vi "TimeForVIPCheck.vi"(8 "error in (no error)":errorcluster) -> (0 "error out":errorcluster, 3 "Check VIP?":bool)   [LabVIEW 2014, in "Raspberry Pi Compatible Compiler for LabVIEW.lvlib" / "GitHub API.lvlib"]
uses:
  GitHub API.lvlib
  RasPi Compiler/Compile and Download App/Custom Controls/Local Setup Parameters.ctl
  Raspberry Pi Compatible Compiler for LabVIEW.lvlib
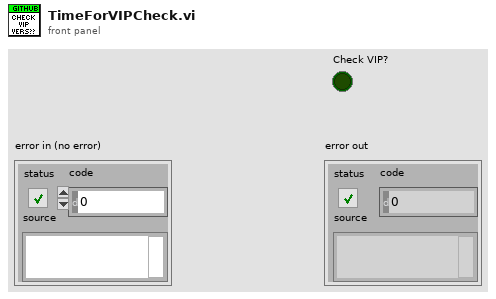
[diagram p1: front panel]
types:
  T1 = typedef "Raspberry Pi Compatible Compiler for LabVIEW.lvlib/Local Setup Parameters.ctl" = enum16{"Add Last VI", "Read Last VI", "Add Board IP", "Remove Board IP", "Read All Board IP", "Add Runtime Version", "Read Runtime Version", "Add Package Version", "Read Package Version", "Add VIPCheck Time", "Read VIPCheck Time"}
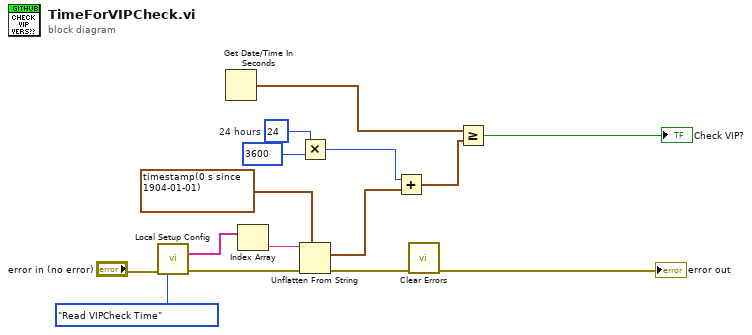
[diagram p0: block diagram]
diagram:
  w1 = 24  # 24 hours
  n1 = call "Local Setup Config.vi"("Local Setup Param"=Local_Setup_Parameters."Read VIPCheck Time", "error in"="error in (no error)") -> ("KeyValues"=w13:string[], "error out"=w12:errorcluster)  [unwired: 10 in, 2 out]
  n2 = Get Date/Time In Seconds() -> (seconds since 1Jan1904=w5:timestamp)
  n3 = Index Array(array=w13) -> (element=w11:string)  [unwired: 1 in]
  n4 = Multiply(x=w1, y=3600) -> (x*y=w2:i32)
  n5 = Unflatten From String(type=timestamp(0 s since 1904-01-01) ("Time Stamp"), binary string=w11, error in (no error)=w12) -> (value=w7:timestamp, error out=w9:errorcluster)  [unwired: 2 in, 1 out]
  n6 = Add(x=w2, y=w7) -> (x+y=w4:timestamp)
  n7 = call <vilib>:"Clear Errors.vi"("error in (no error)"=w9) -> ("error out"=→"error out":errorcluster)  [unwired: 5 in, 1 out]
  n8 = Greater Or Equal?(x=w5, y=w4) -> (x >= y?=→"Check VIP?":bool)
